vi "save scanivalve config file.vi"(10 "file path":path, 11 "scanivalveChannels":T1[][](array[typedef])) -> ()   [LabVIEW 2018]
uses:
  type defs/scanivalve channel control.ctl
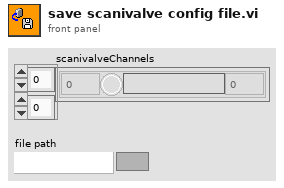
[diagram p1: front panel]
types:
  T1 = typedef "scanivalve channel control.ctl" = cluster{"port":u16, "active":bool, "channelName":string, "range":dbl}
  T2 = enum16{"open", "replace", "create", "open or create", "replace or create", "replace or create with confirmation"}
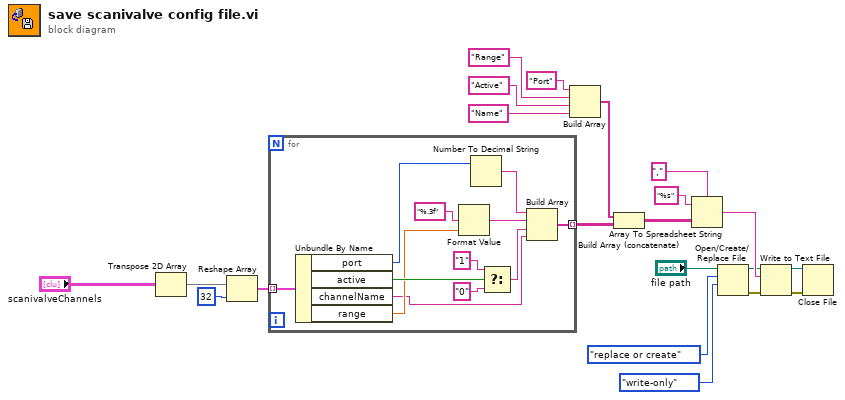
[diagram p0: block diagram]
diagram:
  n1 = Transpose 2D Array(2D array="scanivalveChannels") -> (transposed array=w2:T1[][])
  n2 = Reshape Array(w2, 32 ("dimension size")) -> (w4:T1[])
  n3 = for {
    tunnel: w4 -> [w33] mode=indexing
    tunnel: [w25] -> w9 mode=indexing
    n4 = Unbundle By Name(w33) -> ("port"=w32:u16, "active"=w31:bool, "channelName"=w22:string, "range"=w28:dbl)
    n5 = Format Value(format string="%.3f", value (0)=w28) -> (output string=w24:string)  [unwired: 1 in]
    n6 = Number To Decimal String(number=w32) -> (decimal integer string=w26:string)  [unwired: 1 in]
    n7 = Select(t="1", s=w31, f="0") -> (s? t:f=w23:string)
    n8 = Build Array(w26, w24, w23, w22) -> (w25:string[])
  }
  n9 = Build Array("Port" ("format string"), "Range" ("format string"), "Active" ("format string"), "Name" ("format string")) -> (w10:string[])
  n10 = Build Array (concatenate)(w10, w9) -> (w11:string[][])
  n11 = Array To Spreadsheet String(delimiter (Tab)=",", array=w11, 3:"%s" ("format string")) -> (spreadsheet string=w19:string)
  n12 = Open/Create/Replace File(file path (use dialog)="file path", operation (0:open)=T2."replace or create", access (0:read/write)=enum16{"read/write", "read-only", "write-only"}."write-only") -> (refnum out=w18:refnum<file>, error out=w17:errorcluster)  [unwired: 3 in, 1 out]
  n13 = Write to Text File(file (use dialog)=w18, text=w19, error in=w17) -> (refnum out=w21:refnum<file>, error out=w20:errorcluster)  [unwired: 1 in, 1 out]
  n14 = Close File(refnum=w21, error in=w20) -> ()  [unwired: 2 out]
